vi "Main.vi"   [LabVIEW 2018]
doc: "The myRIO Project template acquires acceleration data from the onboard accelerometer and displays the changes of acceleration values in a waveform chart."
uses:
  <vilib>/robotics/Steering/Wheel/Wheel Parameters.ctl
  <vilib>/robotics/Steering/Wheel/Rotation Direction.ctl
  <vilib>/robotics/Steering/Omnidirectional Wheel/NI_Robotics_Omnidirectional Wheel.lvclass
  C:/Program Files (x86)/National Instruments/LabVIEW 2018/vi.lib/robotics/Steering/Wheel/NI_Robotics_Wheel.lvclass
  <vilib>/robotics/Steering/Omnidirectional Wheel/Create Omnidirectional Wheel.vi
  <vilib>/robotics/Steering/Steering Frame/Create User Defined Steering Frame.vi
  <vilib>/robotics/Steering/Create Steering Frame/NI_Robotics_Create Steering Frame.xnode
  <vilib>/robotics/Steering/Steering Frame/NI_Robotics_Steering Frame.lvclass
  <vilib>/robotics/Steering/Class Type Definitions/Steering Frame.ctl
  <vilib>/robotics/Steering/Class Type Definitions/NI_Robotics_Steering Class Types.lvlib
  <vilib>/robotics/Steering/Wheel/NI_Robotics_Wheel.lvclass
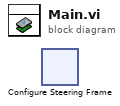
[diagram p0: block diagram]
diagram:
  n1 = xnode ("Configure Steering Frame")() -> ()  [unwired: 1 in, 2 out]
